vi "Read wrapnum.vi"(8 "error in (no error)":errorcluster, 11 "Wrapnum.lvclass in":refnum<class "Wrapnum.lvclass">) -> (0 "error out":errorcluster, 2 "wrapnum":T1, 3 "Wrapnum.lvclass out":refnum<class "Wrapnum.lvclass">)   [LabVIEW 2010, in "TCS.lvlib" / "TCSDataDefinitions.lvlib" / "TCSCommand.lvlib" / "Wrapnum.lvclass"]
uses:
  Wrapnum.lvclass
  Enumerations/WrapnumTypes.ctl
  Wrapnum.lvclass/Wrapnum.ctl
  TCSCommand.lvlib
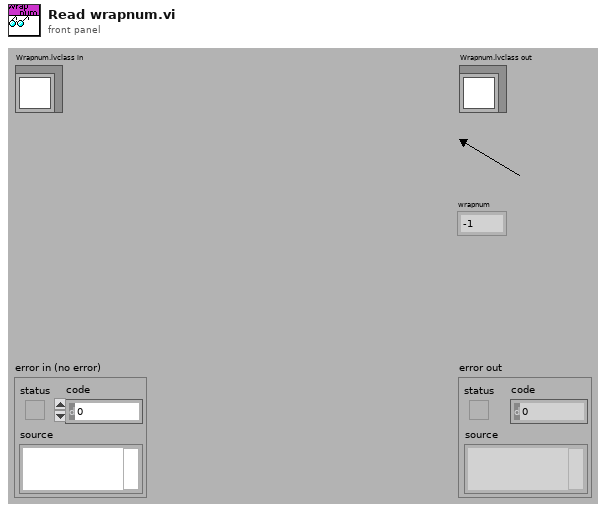
[diagram p1: front panel]
types:
  T1 = typedef "TCS.lvlib/TCSDataDefinitions.lvlib/TCSCommand.lvlib/WrapnumTypes.ctl" = enum16{"-1", "0", "1"}
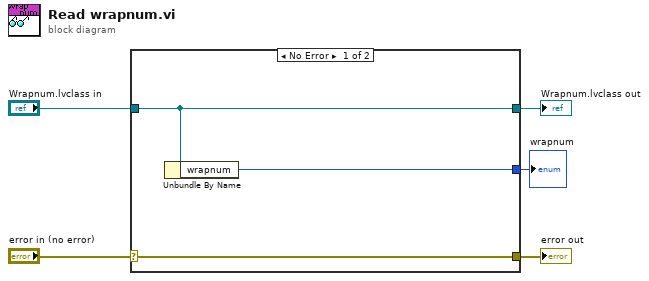
[diagram p0: block diagram]
diagram:
  n1 = case shown="No Error" "error in (no error)" {
    selector: "error in (no error)" -> [w8 w9]
    tunnel: [w8 w9] -> w4
    tunnel: [w7 w10] -> w2
    tunnel: "Wrapnum.lvclass in" -> [w7 w10]
    tunnel: [w6 _] -> w1
    frame No Error {
      n2 = Unbundle By Name(w7) -> ("wrapnum"=w6:T1)
    }
    frame Error {
    }
  }
  "error out" <- w4
  "Wrapnum.lvclass out" <- w2
  "wrapnum" <- w1
